vi "UDP Action Engine.vi"(7 "UDP Action Engine States":T1, 8 "error in (no error)":errorcluster) -> (0 "error out":errorcluster)   [LabVIEW 2016, in "Assert API Components.lvlib" / "Log Assert Core.lvlib"]
doc: "Action engine to open and maintain a UDP reference purely for the purposes of broadcasting the IP of the assert - will be closed down and not used once there is a valid TCP link in place."
uses:
  Log Assert Core.lvlib
  UDP Action Engine States.ctl
  <vilib>/Utility/tcp.llb/UDP Multicast Write-Only Open.vi
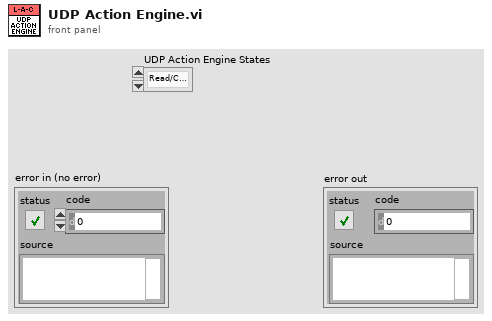
[diagram p1: front panel]
types:
  T1 = typedef "Assert API Components.lvlib/Log Assert Core.lvlib/UDP Action Engine States.ctl" = enum16{"Read/Create UDP", "Broadcast IP", "Close"}
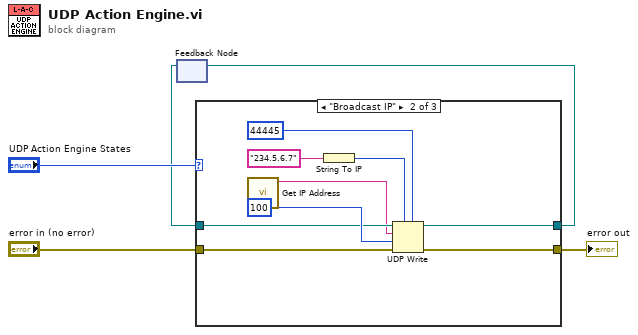
[diagram p0: block diagram]
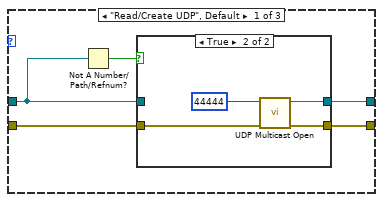
[diagram p2: hidden frame]
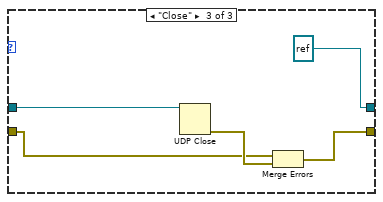
[diagram p4: hidden frame]
diagram:
  n1 = feedback #1() -> (w3:refnum<k16>)  [unwired: 1 in]
  n2 = case shown="\"Broadcast IP\"" "UDP Action Engine States" {
    tunnel: [w10 w20 refnum<k16> refnum ("connection ID out")] -> w4
    tunnel: w3 -> [w6 w21 w30]
    tunnel: "error in (no error)" -> [w9 w22 w26]
    tunnel: [w8 w19 w27] -> w1
    frame "Read/Create UDP", Default {
      n3 = Not A Number/Path/Refnum?(number/path/refnum=w6) -> (NaN/Path/Refnum?=w7:bool)
      n4 = case shown="True" w7 {
        tunnel: [w12 w15] -> w10
        tunnel: w9 -> [w11 w14]
        tunnel: [w11 w13] -> w8
        tunnel: w6 -> [w12 _]
        frame False {
        }
        frame True {
          n5 = call-poly <vilib>:"UDP Multicast Open.vi"("error in (no error)"=w14, "port"=u16 44444) -> ("error out"=w13:errorcluster, "connection ID"=w15:refnum<k16>)  [unwired: 8 in]
        }
      }
    }
    frame "Broadcast IP" {
      n6 = call "Get IP Address.vi"() -> ("IP Address"=w17:string)  [unwired: 11 in]
      n7 = String To IP(1:"234.5.6.7" ("name")) -> (0:w24:u32)
      n8 = UDP Write(address=w24, port or service name=u16 44445, connection ID=w21, data in=w17, 8:w22, 9:100 ("timeout ms (25000)")) -> (error out=w19:errorcluster, 3:w20:refnum<k16>)
    }
    frame "Close" {
      n9 = UDP Close(connection ID=w30) -> (error out=w28:errorcluster)  [unwired: 1 in, 1 out]
      n10 = Merge Errors(w26, w28) -> (w27:errorcluster)
    }
  }
  "error out" <- w1
  n11 = feedback-in #1(w4) -> ()
